vi "Meas Result Remove Readings.vi"(7 "ids of selected":i32[](array[numeric]), 8 "error in":errorcluster, 9 "sweep spot index":u16, 11 "result":T1) -> (0 "error out":errorcluster, 3 "result out":T1)   [LabVIEW 2020]
doc: "Removes selected readings from result data."
uses:
  Meas Results.ctl
  bridge/Bridge Frequency Readings Data.ctl
  drivers/TWM client/Meas Proc QWTB Spectrum Data.ctl
  drivers/TWM client/TWM Phase Info.ctl
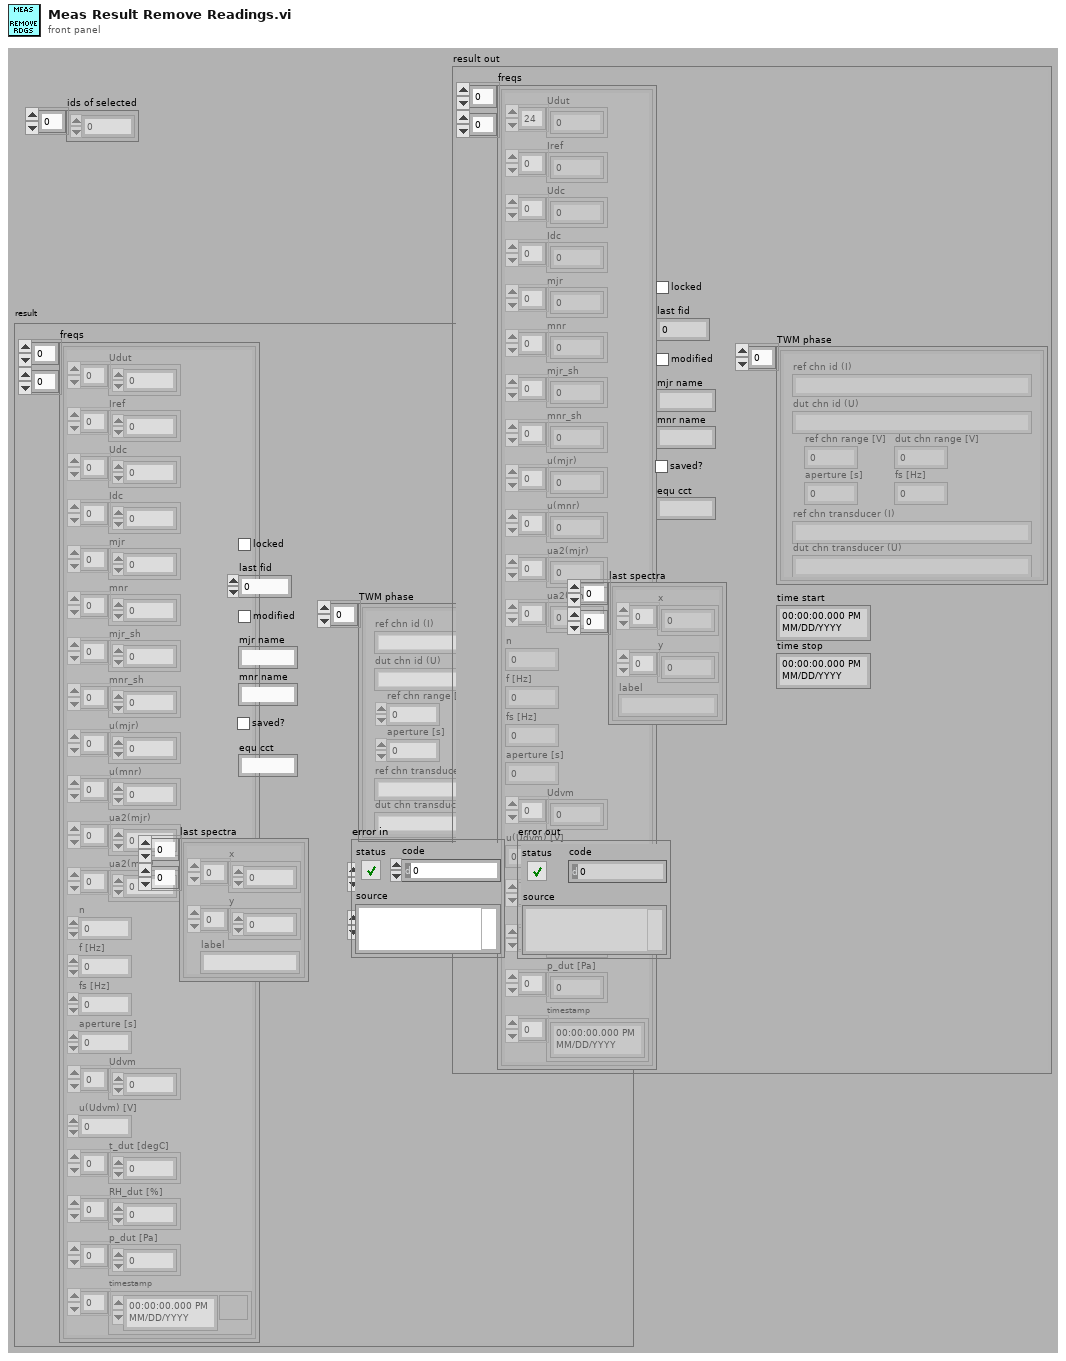
[diagram p1: front panel]
types:
  T1 = typedef "Meas Results.ctl" = cluster{"freqs":T2[][], "locked":bool, "last fid":i32, "modified":bool, "mjr name":string, "mnr name":string, "last spectra":T3[][], "saved?":bool, "TWM phase":T4[], "time start":timestamp, "time stop":timestamp, "equ cct":string}
  T2 = typedef "Bridge Frequency Readings Data.ctl" = cluster{"Udut":dbl[], "Iref":dbl[], "Udc":dbl[], "Idc":dbl[], "mjr":dbl[], "mnr":dbl[], "mjr_sh":dbl[], "mnr_sh":dbl[], "u(mjr)":dbl[], "u(mnr)":dbl[], "ua2(mjr)":dbl[], "ua2(mnr)":dbl[], "n":i32, "f [Hz]":dbl, "fs [Hz]":dbl, "aperture [s]":dbl, "Udvm":dbl[], "u(Udvm) [V]":dbl, "t_dut [degC]":dbl[], "RH_dut [%]":dbl[], "p_dut [Pa]":dbl[], "timestamp":timestamp[]}
  T3 = typedef "Meas Proc QWTB Spectrum Data.ctl" = cluster{"x":sgl[], "y":sgl[], "label":string}
  T4 = typedef "TWM Phase Info.ctl" = cluster{"ref chn id (I)":string, "dut chn id (U)":string, "ref chn range [V]":dbl, "dut chn range [V]":dbl, "aperture [s]":dbl, "fs [Hz]":dbl, "ref chn transducer (I)":string, "dut chn transducer (U)":string}
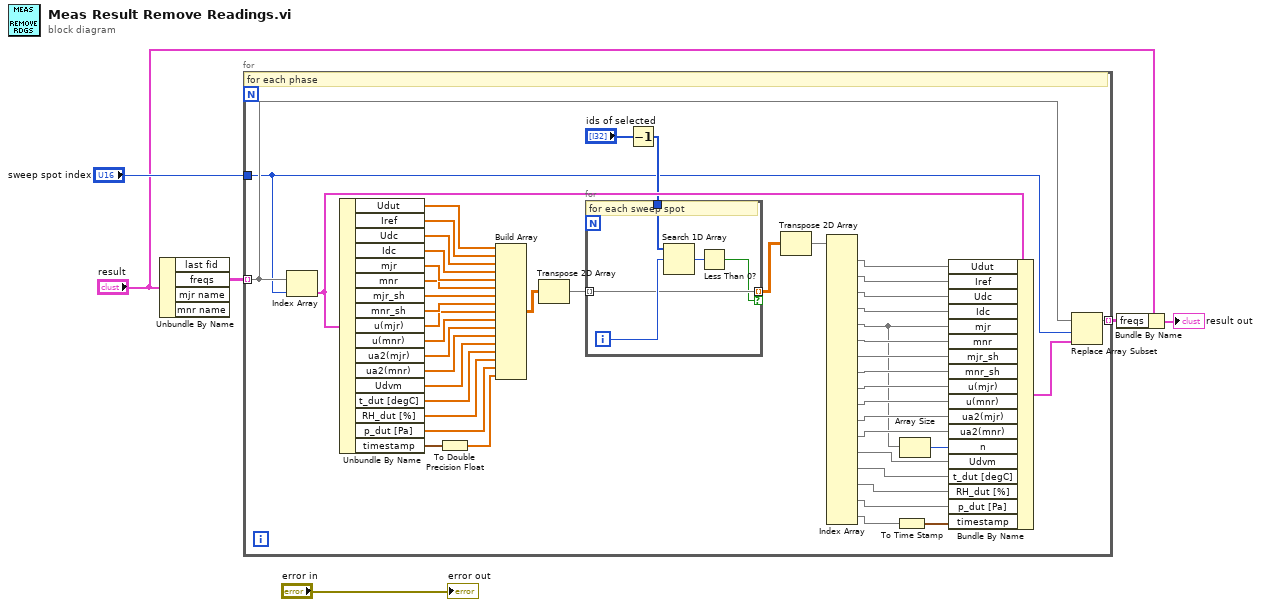
[diagram p0: block diagram]
diagram:
  n1 = Unbundle By Name("result") -> ("freqs"=w6:T2[][])  [unwired: 3 out]
  n2 = for {
    tunnel: w6 -> [w25] mode=indexing
    tunnel: "sweep spot index" -> [w11]
    tunnel: [w21] -> w3 mode=indexing
    # "for each phase"
    n3 = Index Array(array=w25, index=w11) -> (element=w37:T2)
    n4 = Unbundle By Name(w37) -> ("Udut"=w54:dbl[], "Iref"=w53:dbl[], "Udc"=w52:dbl[], "Idc"=w51:dbl[], "mjr"=w50:dbl[], "mnr"=w49:dbl[], "mjr_sh"=w48:dbl[], "mnr_sh"=w47:dbl[], "u(mjr)"=w46:dbl[], "u(mnr)"=w45:dbl[], "ua2(mjr)"=w44:dbl[], "ua2(mnr)"=w43:dbl[], "Udvm"=w19:dbl[], "t_dut [degC]"=w17:dbl[], "RH_dut [%]"=w16:dbl[], "p_dut [Pa]"=w15:dbl[], "timestamp"=w10:timestamp[])
    n5 = To Double Precision Float(number=w10) -> (double precision float=w9:dbl[])
    n6 = Build Array(w54, w53, w52, w51, w50, w49, w48, w47, w46, w45, w44, w43, w19, w17, w16, w15, w9) -> (w42:dbl[][])
    n7 = Transpose 2D Array(2D array=w42) -> (transposed array=w41:dbl[][])
    n8 = Decrement(x="ids of selected") -> (x-1=w20:i32[])
    n9 = for {
      tunnel: w41 -> [w57] mode=indexing
      tunnel: w20 -> [w59]
      tunnel: [w57] -> w39 mode=indexing if=w55
      i -> [w58]
      # "for each sweep spot"
      n10 = Search 1D Array(1D array=w59, element=w58) -> (index of element=w56:i32)  [unwired: 1 in]
      n11 = Less Than 0?(x=w56) -> (x < 0?=w55:bool)
    }
    n12 = Transpose 2D Array(2D array=w39) -> (transposed array=w38:dbl[][])
    n13 = Index Array(array=w38) -> (element #1=w36:dbl[], element #2=w35:dbl[], element #3=w34:dbl[], element #4=w33:dbl[], element #5=w22:dbl[], element #6=w32:dbl[], element #7=w31:dbl[], element #8=w30:dbl[], element #9=w29:dbl[], element #10=w28:dbl[], element #11=w27:dbl[], element #12=w23:dbl[], element #13=w18:dbl[], element #14=w14:dbl[], element #15=w13:dbl[], element #16=w12:dbl[], element #17=w8:dbl[])  [unwired: 34 in]
    n14 = To Time Stamp(1:w8) -> (0:w7:timestamp[])
    n15 = Array Size(array=w22) -> (size(s)=w24:i32)
    n16 = Bundle By Name(cluster=w37, "Udut"=w36, "Iref"=w35, "Udc"=w34, "Idc"=w33, "mjr"=w22, "mnr"=w32, "mjr_sh"=w31, "mnr_sh"=w30, "u(mjr)"=w29, "u(mnr)"=w28, "ua2(mjr)"=w27, "ua2(mnr)"=w23, "n"=w24, "Udvm"=w18, "t_dut [degC]"=w14, "RH_dut [%]"=w13, "p_dut [Pa]"=w12, "timestamp"=w7) -> (w26:T2)
    n17 = Replace Array Subset(array=w25, new element=w26, index=w11) -> (w21:T2[])
  }
  n18 = Bundle By Name(cluster="result", "freqs"=w3) -> (→"result out":T1)
  "error out" <- "error in"
